vi "heartBeatRead.vi"(8 "error in (no error)":errorcluster, 9 "heartbeat object in":refnum<k20>, 11 "MotorController in":refnum<class "MotorController.lvclass">) -> (0 "error out":errorcluster, 1 "heartbeat object out":refnum<k20>, 3 "MotorController out":refnum<class "MotorController.lvclass">)   [LabVIEW 2017, in "MotorController.lvclass"]
uses:
  MotorController.lvclass
  MotorController.lvclass/MotorController.ctl
  <vilib>/CANopenLib/CANOPEN.llb/CANopen Heartbeat State Read.vi
panel:
  out "timestamp":timestamp
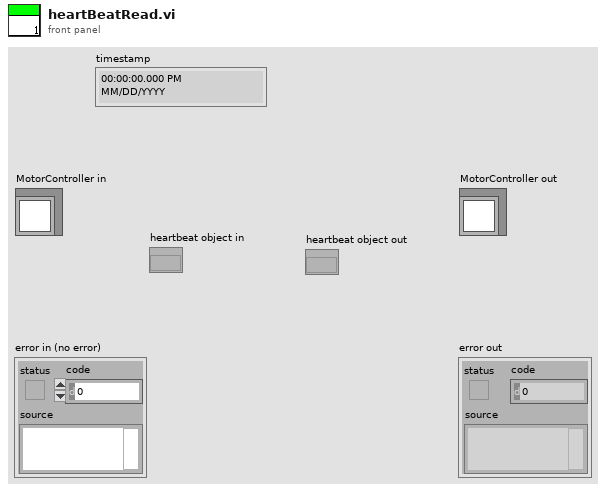
[diagram p1: front panel]
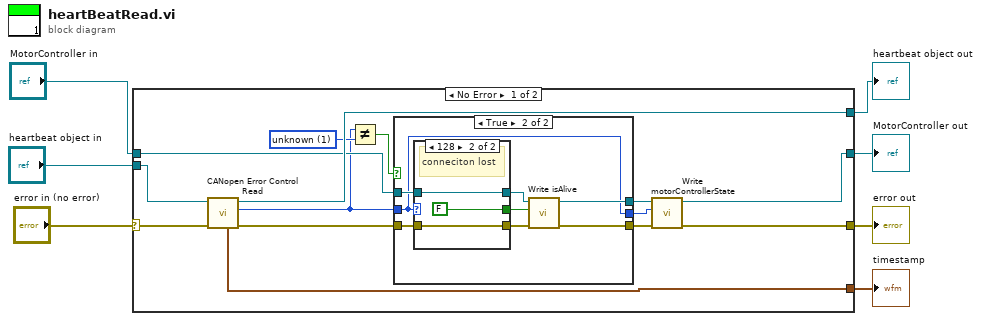
[diagram p0: block diagram]
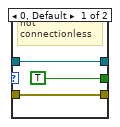
[diagram p3: hidden frame]
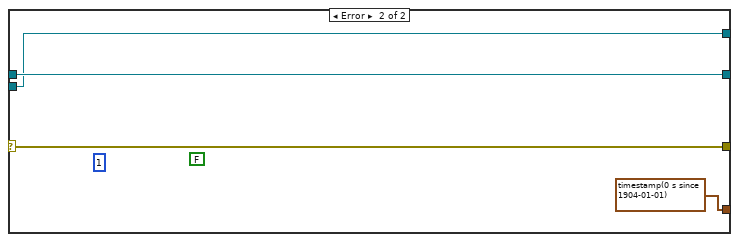
[diagram p4: hidden frame]
diagram:
  n1 = case shown="No Error" "error in (no error)" {
    selector: "error in (no error)" -> [w21 w42]
    tunnel: [w10 w42] -> w6
    tunnel: [w13 w41] -> w4
    tunnel: "MotorController in" -> [w16 w41]
    tunnel: "heartbeat object in" -> [w20 w40]
    tunnel: [w19 w40] -> w2
    tunnel: [w18 timestamp(0 s since 1904-01-01) ("timestamp")] -> w1
    frame No Error {
      w9 = u16 1 items=["unknown"=1, "bootup"=0, "stopped"=4, "operational"=5, "pre-operational"=127, "connection lost"=128] ("state")
      n2 = call-poly <vilib>:"CANopen Error Control Read.vi"("error in (no error)"=w21, "heartbeat object in"=w20) -> ("error out"=w15:errorcluster, "state"=w8:u16, "heartbeat object out"=w19:refnum<k20>, "timestamp"=w18:timestamp)  [unwired: 6 in]
      n3 = Not Equal?(x=w8, y=w9) -> (x != y?=w17:bool)
      n4 = case shown="True" w17 {
        tunnel: w16 -> [w24 w31]
        tunnel: w8 -> [w22 w25]
        tunnel: w15 -> [w23 w29]
        tunnel: [w24 w27] -> w14
        tunnel: [w23 w26] -> w11
        tunnel: [w22 w25] -> w12
        frame False {
        }
        frame True {
          n5 = case shown="128" w25 {
            tunnel: [TRUE ("isAlive") FALSE ("isAlive")] -> w32
            tunnel: w31 -> [w35 w37]
            tunnel: [w35 w37] -> w30
            tunnel: w29 -> [w33 w36]
            tunnel: [w33 w36] -> w28
            frame 0, Default {
              # "not connectionless"
            }
            frame 128 {
              # "conneciton lost"
            }
          }
          n6 = call "Write isAlive.vi"("error in (no error)"=w28, "isAlive"=w32, "MotorController in"=w30) -> ("error out"=w26:errorcluster, "MotorController out"=w27:refnum<class "MotorController.lvclass">)  [unwired: 7 in]
        }
      }
      n7 = call "Write motorControllerState.vi"("error in (no error)"=w11, "motorControllerState"=w12, "MotorController in"=w14) -> ("error out"=w10:errorcluster, "MotorController out"=w13:refnum<class "MotorController.lvclass">)  [unwired: 7 in]
    }
    frame Error {
      (unwired) FALSE
      (unwired) u16 1 ("state")
    }
  }
  "error out" <- w6
  "MotorController out" <- w4
  "heartbeat object out" <- w2
  "timestamp" <- w1
